vi "VariantToString.vi"(0 "Variant":variant, 1 "Binary floats?":bool caption="Binary floats? (F)", 5 "Float precision":i16=20 caption="Float precision (20)", 7 "Radix point":T1=enum."Period (.)" caption="Radix point (.)", 9 "Remove trailing zeroes?":bool=TRUE caption="Remove trailing zeroes? (T)", 11 "Error in":errorcluster caption="Error in (no error)") -> (4 "Name":string, 6 "Type":string, 8 "Labels":string[](array[string]), 10 "Values":string[](array[string]), 15 "Error out":errorcluster)   [LabVIEW 2017, in "GPString.lvlib"]
doc: "Converts <B>Variant</B> to a string representation as <B>Name</B>, <B>Type</B>, <B>Labels</B> and <B>Values</B>.\n\n<B>Extended parsing</B>\nSome <B>Type</B>s will feature extended parsing with human readable strings output in <B>Labels</B> and <B>Values</B>. Types with such extended parsing are:\n\n- Booleans\n- Numbers (ints, real and complex floats, fixed-point values)\n- Enums\n- Strings\n- Paths\n- Timestamps\n- Refnums\n- Arrays of any of the above\n\nA few examples of types with extended parsing:\n\n<B>Name</B> = <name>\n<B>Type</B> = \"SGL\"\n<B>Labels</B> = \"Value\"\n<B>Values</B> = \"-7.550602\"\n\n<B>Name</B> = <name>\n<B>Type</B> = \"Enum U8\"\n<B>Labels</B> = \"Items\" ; \"Value\"\n<B>Values</B> = \"[\"One\",\"Two\",\"Three\",\"Four\"]\" ; \"Three\"\n\n<B>Name</B> = <name>\n<B>Type</B> = \"Array\"\n<B>Labels</B> = \"ArrayType\" ; \"Values\"\n<B>Values</B> = \"SGL\" ; \"[[11.2,-9.003][0.01,84.45][-3.7,11.966455]]\"\n\n<B>Name</B> = <name>\n<B>Type</B> = \"Array\"\n<B>Labels</B> = \"ArrayType\" ; \"Items\" ; \"Values\"\n<B>Values</B> = \"Enum U8\" ; \"[\"One\",\"Two\",\"Three\",\"Four\"]\" ; \"[\"Two\",\"Four\"]\"\n\n<B>Binary form</B>\nOther LabVIEW data types will be output in binary form like this:\n\n<B>Name</B> = <name>\n<B>Type</B> = \"Variant\"\n<B>Labels</B> = \"Value\"\n<B>Values</B> = <flattened string of <B>Variant</B>>\n\nThe binary form still lets you use the data in serialized form, e.g. to write it to an ASCII file, read it back, and convert it succesfully into the original <B>Variant</B>. It will just not be in human readable/editable form. Currently binary types are:\n\n- Classes\n- Data (digital, express, external)\n- Floats with units\n- Pictures\n- Variants\n- Waveforms\n- Arrays of any of the above\n\n<B>Floating point numbers</B>\nFor when <B>Variant</B> contains floating point numbers you can optionally specify their conversion to string:\n\n<B>Binary floats?</B> if set to True encodes floating point values as hexadecimal strings guaranteeing full precision. The default is to encode floats as ASCII strings.\n\nIf floats are encoded as ASCII strings <B>Float precision</B>, <B>Radix point</B>, and <B>Remove trailing zeroes?</B> lets you specify their encoding. Note that floating point numbers risk precision loss if they are converted to and from string representation with too few digits.\n\n<B>Radix point</B> doubles as a selector for array element separator character in strings. <B>Radix point</B> = \".\" infers array element separator charactor \",\" (comma), while <B>Radix point</B> = \",\" infers array element separator charactor \";\" (semicolon).\n\n<B>Clusters</B>\nClusters are encoded with each element in either extended parsing or binary form depending on the type of each embedded element. Clusters will be output like this:\n\n<B>Name</B> = <name>\n<B>Type</B> = \"Cluster\"\n<B>Labels</B> = \"Names\" ; <element 1 labels>...<element n labels>\n<B>Values</B> = \"[<element 1 name>...<element n name>]\" ; <element 1 values>...<element n values>\n\nEach sub-element in the cluster will be labeled in dot-notation following the data hierarchy within the cluster. An example of a cluster named \"Top\" containing a single element (name: \"MyNumber\", type: I32, value: 9):\n\n<B>Name</B> = \"Top\"\n<B>Type</B> = \"Cluster\"\n<B>Labels</B> = \"Names\" ; \"MyNumber.Name\" ; \"MyNumber.Type\" ; \"MyNumber.Value\"\n<B>Values</B> = \"[\"MyNumber\"]\" ; \"MyNumber\" ; \"I32\" ; \"9\"\n\nThis VI is inlined and it runs only if there is no error on <B>Error in</B>.\n\nSteen Schmidt\nGPower\n28/9 2015"
uses:
  GPString.lvlib
  Typedefs/RadixPoint.ctl
panel:
  # "Copyright © 2015\nGPower\nSee enclosed license file for terms and conditions"
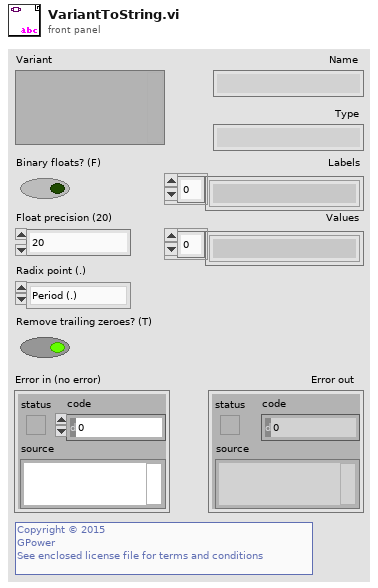
[diagram p1: front panel]
types:
  T1 = typedef "GPString.lvlib/RadixPoint.ctl" = enum16{"System", "Period (.)", "Comma (,)"}
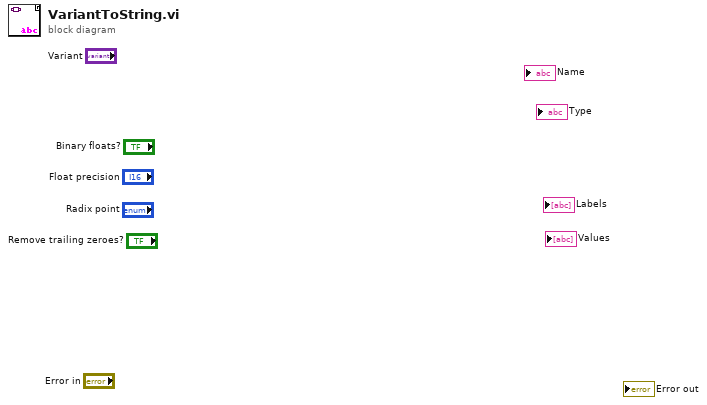
[diagram p0: block diagram]
diagram:
